vi "RSD Responce Parse.vi"(7 "Checksum used":bool=TRUE, 11 "Responce":string) -> (0 "Checksum":string, 1 "Value (decimal)":u32, 2 "Value (string)":string, 3 "OK":string, 4 "Command":string, 5 "STX":string, 6 "Address":string)   [LabVIEW 2016, in "Samwontech TEMP2xxx.lvlib"]
uses:
  Samwontech TEMP2xxx.lvlib
panel:
  in  "Count number (only 1 support now)":u8=1
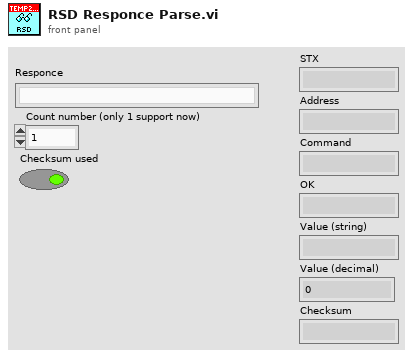
[diagram p1: front panel]
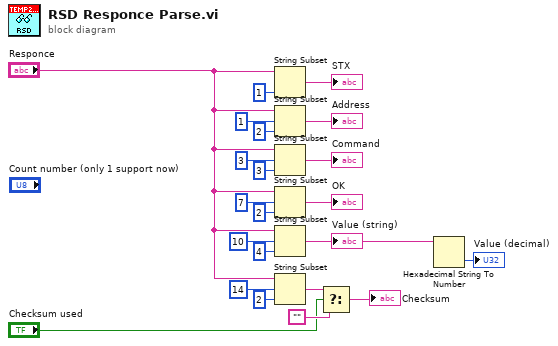
[diagram p0: block diagram]
diagram:
  n1 = String Subset(string="Responce", length (rest)=1 ("length (rest)")) -> (substring=→"STX":string)  [unwired: 1 in]
  n2 = String Subset(string="Responce", offset (0)=1 ("length (rest)"), length (rest)=2 ("length (rest)")) -> (substring=→"Address":string)
  n3 = String Subset(string="Responce", offset (0)=3 ("length (rest)"), length (rest)=3 ("length (rest)")) -> (substring=→"Command":string)
  n4 = String Subset(string="Responce", offset (0)=7 ("length (rest)"), length (rest)=2 ("length (rest)")) -> (substring=→"OK":string)
  n5 = String Subset(string="Responce", offset (0)=10 ("length (rest)"), length (rest)=4 ("length (rest)")) -> (substring=w9:string)
  "Value (string)" <- w9
  n6 = String Subset(string="Responce", offset (0)=14 ("length (rest)"), length (rest)=2 ("length (rest)")) -> (substring=w4:string)
  n7 = Select(t=w4, s="Checksum used", f="") -> (s? t:f=→"Checksum":string)
  n8 = Hexadecimal String To Number(string=w9) -> (number=→"Value (decimal)":u32)  [unwired: 2 in, 1 out]
